vi "While-loop-wait-sample.vi"() -> ()   [LabVIEW 2020]
panel:
  out "Seconds":dbl
  in  "stop\nloop":bool
  out "Loop\nCount":i32
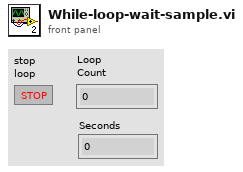
[diagram p1: front panel]
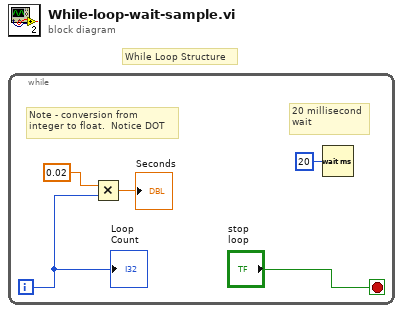
[diagram p0: block diagram]
diagram:
  # "While Loop Structure"
  n1 = while {
    i -> [w3]
    stop <- "stop\nloop" stop-if-true
    # "20 millisecond\nwait"
    # "Note - conversion from\ninteger to float.  Notice DOT"
    n2 = Multiply(x=0.02, y=w3) -> (x*y=→"Seconds":dbl)
    n3 = Wait (ms)(milliseconds to wait=u32 20) -> ()  [unwired: 1 out]
    "Loop\nCount" <- w3
  }
